vi "速度子VI1.vi"(0 "脉冲数":i32) -> (1 "分频基数高位":string, 2 "分频基数低位":string)   [LabVIEW 2014]
panel:
  # "Max=65535"
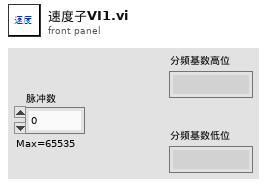
[diagram p1: front panel]
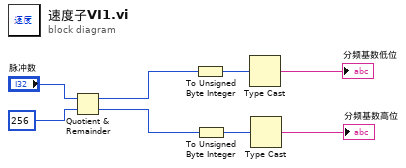
[diagram p0: block diagram]
diagram:
  n1 = Quotient & Remainder(x="脉冲数", y=256) -> (x-y*floor(x/y)=w6:i32, floor(x/y)=w1:i32)
  n2 = To Unsigned Byte Integer(number=w6) -> (unsigned 8bit integer=w5:u8)
  n3 = To Unsigned Byte Integer(number=w1) -> (unsigned 8bit integer=w2:u8)
  n4 = Type Cast(x=w5) -> (*(type *) &x=→"分频基数低位":string)  [unwired: 1 in]
  n5 = Type Cast(x=w2) -> (*(type *) &x=→"分频基数高位":string)  [unwired: 1 in]
